vi "TDMS Reader.vi"() -> ()   [LabVIEW 2018]
panel:
  out "채널 데이터":waveform(dbl)(graph)
  in  "데이터 세트":string(combo)="시간 데이터"
  out "테스트 수행자":string
  out "테스트 시간":timestamp
  in  "시리얼 번호":string
  in  "TDMS 파일 경로":path
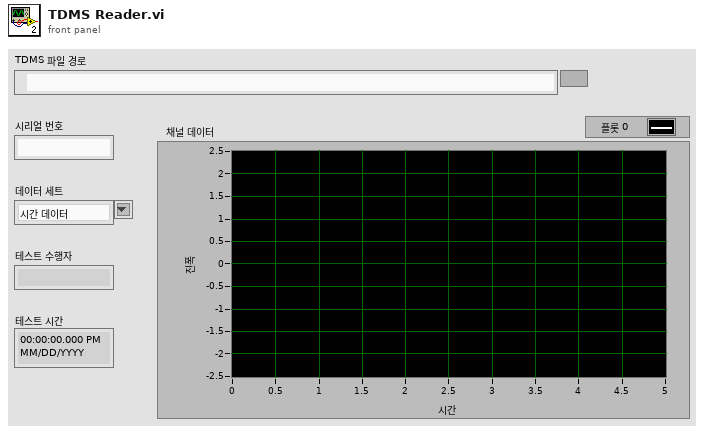
[diagram p1: front panel]
types:
  T1 = enum16{"open", "open or create", "create or replace", "create", "open (read-only)"}
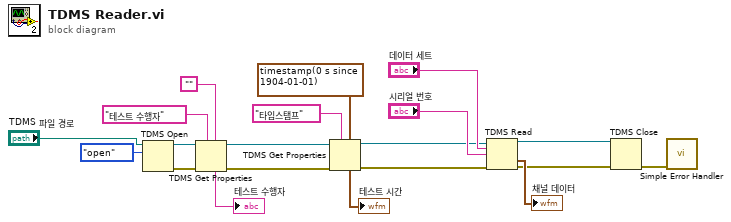
[diagram p0: block diagram]
diagram:
  n1 = TDMS Open(10:T1."open" ("동작(0:open)"), 11:"TDMS 파일 경로") -> (0:w18:errorcluster, 3:w17:refnum<k34>)  [unwired: 5 in]
  n2 = TDMS Get Properties(5:"", 7:"테스트 수행자" ("프로퍼티 이름"), 8:w18, 11:w17) -> (0:w12:errorcluster, 3:w13:refnum<k34>, 4:→"테스트 수행자":string)  [unwired: 2 in, 3 out]
  n3 = TDMS Get Properties(5:timestamp(0 s since 1904-01-01) ("데이터 타입"), 7:"타임스탬프" ("프로퍼티 이름"), 8:w12, 11:w13) -> (0:w6:errorcluster, 3:w5:refnum<k34>, 4:→"테스트 시간":timestamp)  [unwired: 2 in, 3 out]
  n4 = TDMS Read(0:w5, 5:"데이터 세트", 7:"시리얼 번호", 11:w6) -> (4:w3:refnum<k34>, 10:→"채널 데이터":waveform(dbl), 15:w2:errorcluster)  [unwired: 4 in, 3 out]
  n5 = TDMS Close(8:w2, 11:w3) -> (0:w1:errorcluster)  [unwired: 1 out]
  n6 = call <vilib>:"Simple Error Handler.vi"("error in (no error)"=w1) -> ()  [unwired: 4 in, 5 out]
